vi "Get Launch Viewer Property.vi"(8 "error in (no error)":errorcluster, 11 "Item Ref in":T1 format="%.0x") -> (0 "error out":errorcluster, 2 "launch viewer":bool, 3 "Item Ref out":T1 format="%.0x")   [LabVIEW 2020, in "DSF Shared.lvlib"]
uses:
  DSF Shared.lvlib
  <vilib>/NI VeriStand/Custom Device API/Custom Device Item Ref.ctl
  <vilib>/NI VeriStand/Custom Device API/Get Item Property (Boolean).vi
  <vilib>/NI VeriStand/Custom Device API/Custom Device API.lvlib
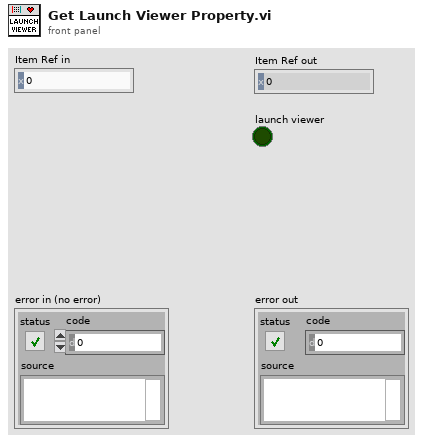
[diagram p1: front panel]
types:
  T1 = typedef "Custom Device API.lvlib/Custom Device Item Ref.ctl" = u64
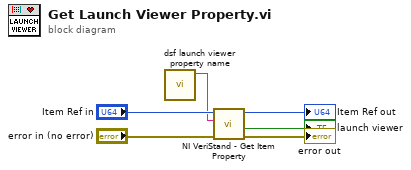
[diagram p0: block diagram]
diagram:
  n1 = call "dsf launch viewer property name.vi"() -> ("launch viewer property name"=w2:string)  [unwired: 11 in]
  n2 = call-poly <vilib>:"NI VeriStand - Get Item Property.vi"("error in (no error)"="error in (no error)", "Property Name"=w2, "Item Ref in"="Item Ref in") -> ("error out"=→"error out":errorcluster, "Value"=→"launch viewer":bool, "Item Ref out"=→"Item Ref out":T1)  [unwired: 5 in, 1 out]
